vi "Depth To Number Channels.vi"(11 "Depth":i32) -> (3 "Channels":i32)   [LabVIEW 2020, in "G-Image.lvlib"]
uses:
  G-Image.lvlib
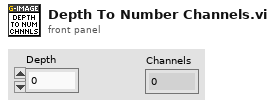
[diagram p1: front panel]
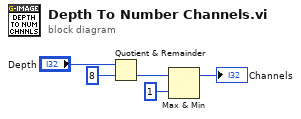
[diagram p0: block diagram]
diagram:
  n1 = Quotient & Remainder(x="Depth", y=8) -> (floor(x/y)=w3:i32)  [unwired: 1 out]
  n2 = Max & Min(x=w3, y=1) -> (max(x,y)=→"Channels":i32)  [unwired: 1 out]
